vi "py-lv-comm_labview-client_jki-sm.vi"() -> ()   [LabVIEW 2016]
uses:
  <vilib>/addons/zeromq/zmq_context.lvclass
  <vilib>/addons/zeromq/zmq_socket.lvclass
panel:
  in  "Tab Control":enum32{"Python Communication", "Debug"}(tab)
  in  "Stop Server":bool
  in  "Connect to Server":bool
  in  "Send Command":bool
  in  "Command":string
  in  "Wait for response":bool=TRUE
  in  "address":string="tcp://127.0.0.1:15213" caption="TCP address of ZMQ server"
  out "Return string":string
  in  "Read Integer":bool
  in  "Read Double":bool
  in  "Read String":bool
  in  "Read Bool":bool
  in  "Read Numpy Array":bool
  in  "Function":string
  in  "Python Property":bool=TRUE
  in  "Arguments":string[](array[string])
  out "int result":i32
  out "double result":dbl
  out "string result":string
  out "bool result":bool
  out "nparray result":dbl[](array[numeric])
  out "Status":string="Idle"
  in  "OK":bool
  out "error":errorcluster
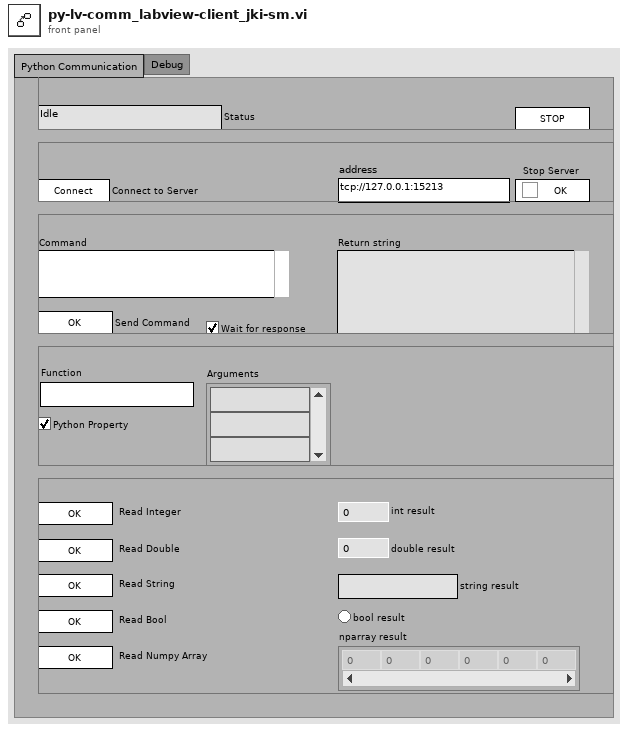
[diagram p1: front panel]
types:
  T1 = enum32{"Invalid", "Standard", "Closed", "Hidden", "Minimized", "Maximized"}
  T2 = enum32{"invalid app kind", "Development System", "Run Time System", "Student Edition", "Embedded LabVIEW", "Evaluation", "Custom"}
  T3 = cluster{"Core":cluster{"Current VI Reference":refnum<vi>, "Close Panel on Exit?":bool}, "zmq_context":refnum<class "zmq_context.lvclass">, "zmq_socket":refnum<class "zmq_socket.lvclass">, "Function":string, "Arguments":string[], "Python Property":bool, "return string":string}
  T4 = cluster{"Current VI Reference":refnum<vi>, "Close Panel on Exit?":bool}
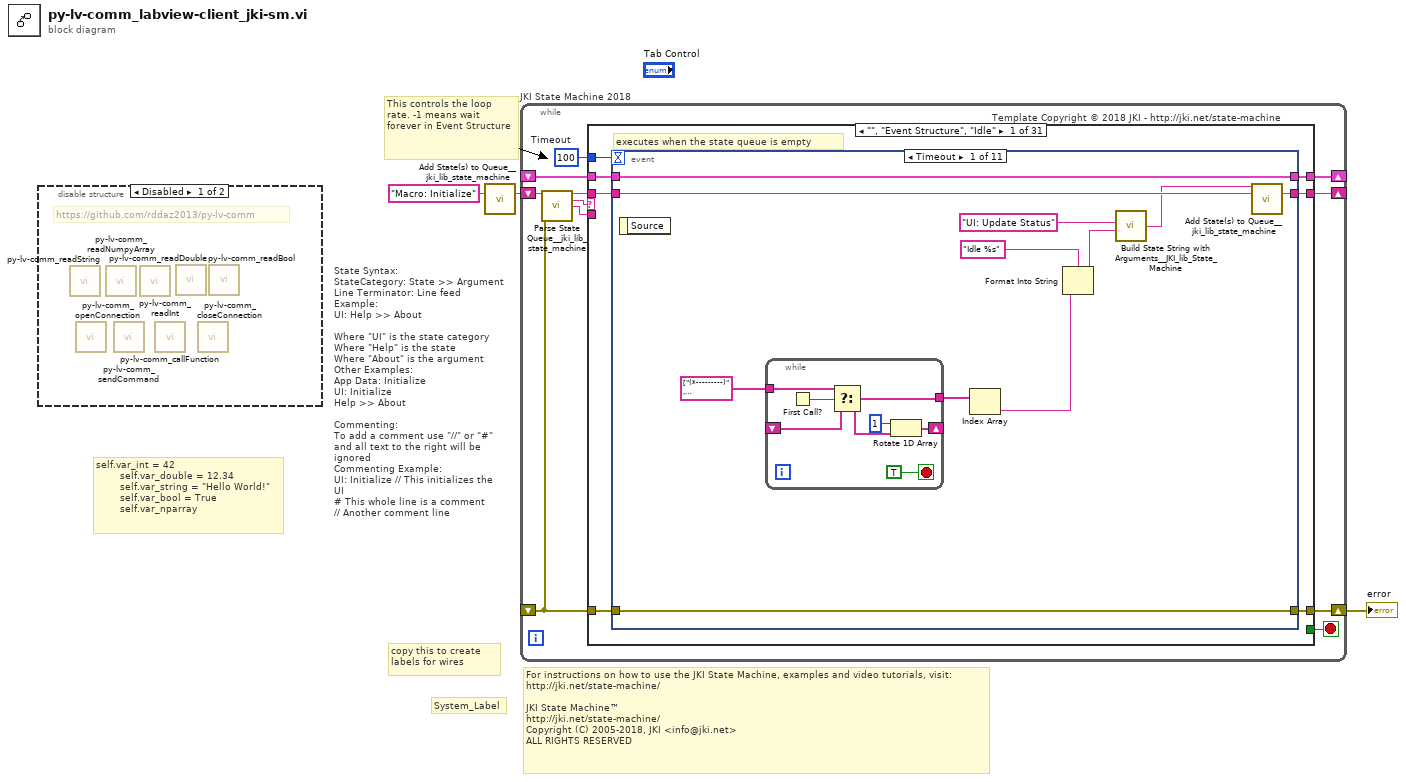
[diagram p0: block diagram]
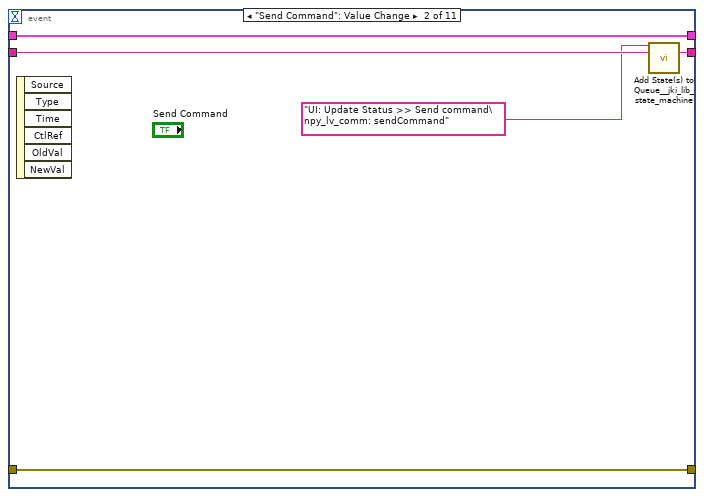
[diagram p3: hidden frame]
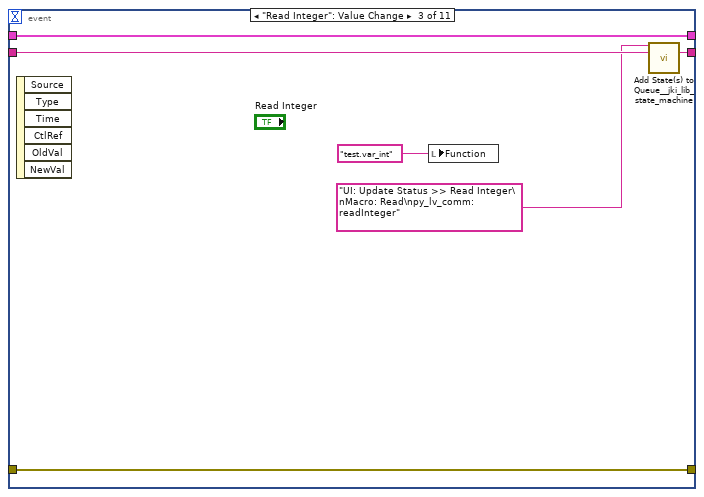
[diagram p4: hidden frame]
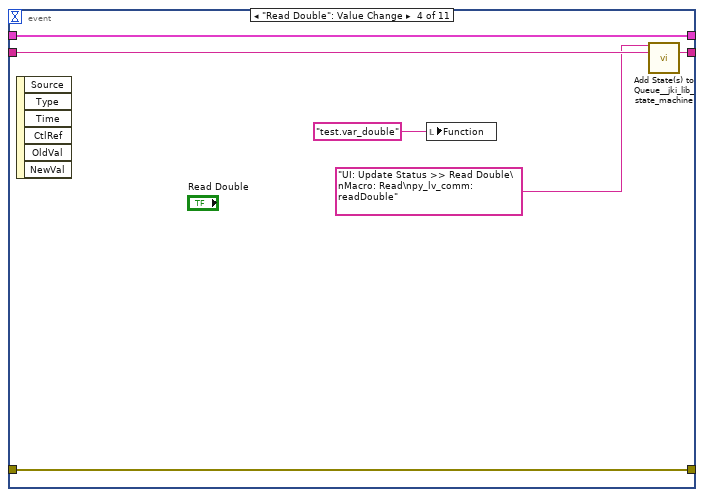
[diagram p5: hidden frame]
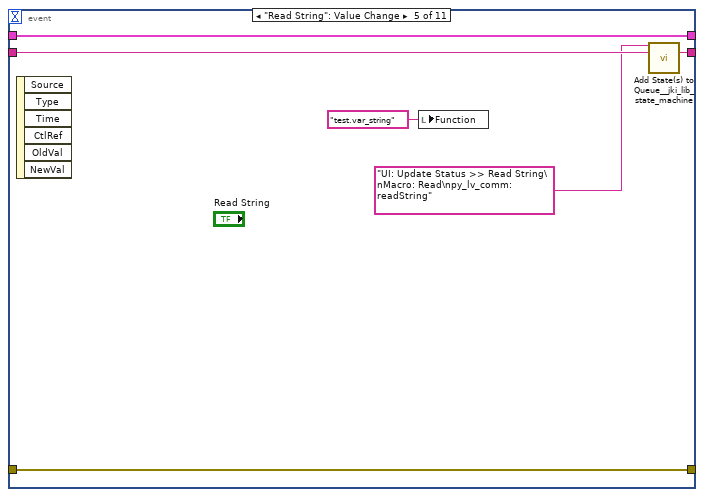
[diagram p6: hidden frame]
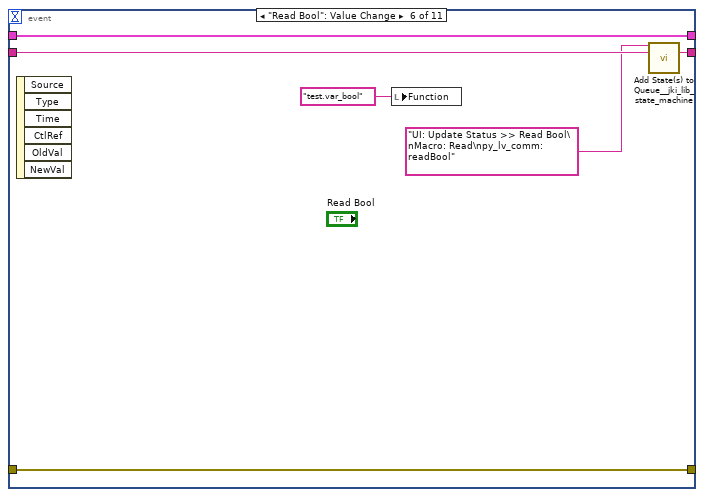
[diagram p7: hidden frame]
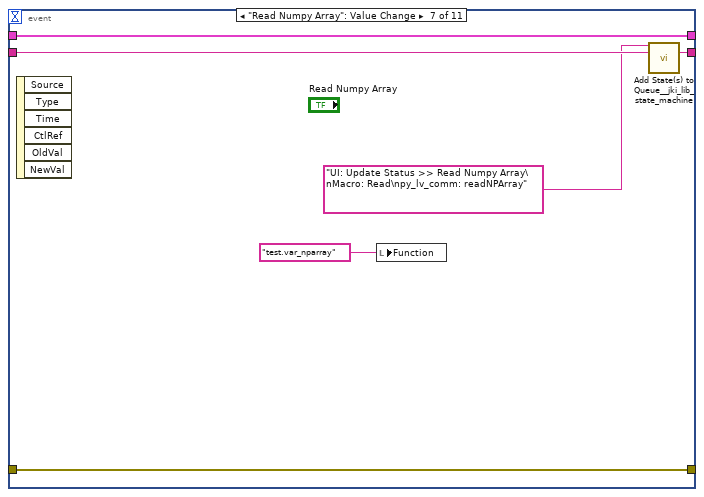
[diagram p8: hidden frame]
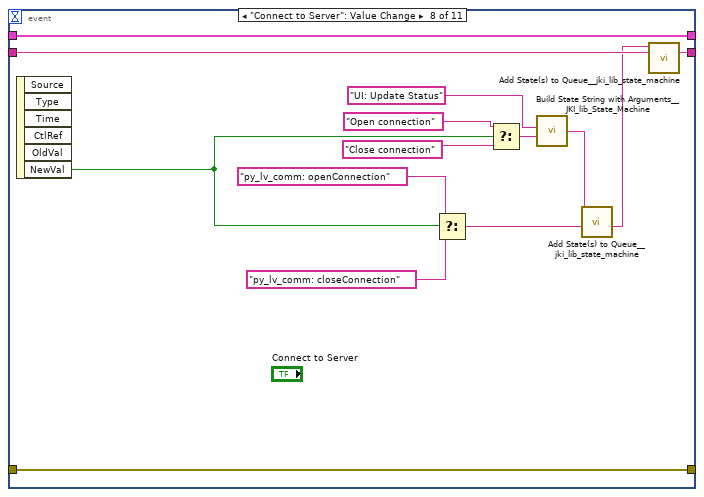
[diagram p9: hidden frame]
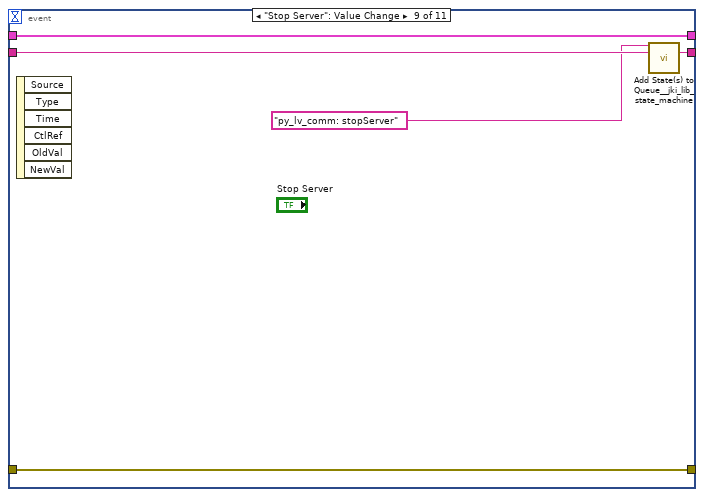
[diagram p10: hidden frame]
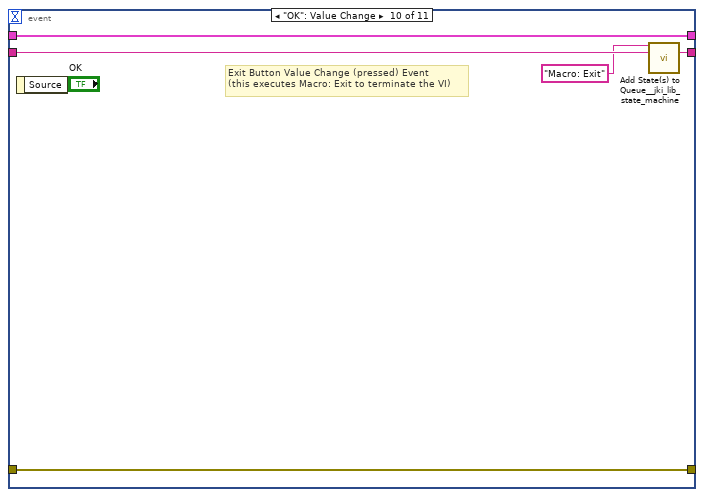
[diagram p11: hidden frame]
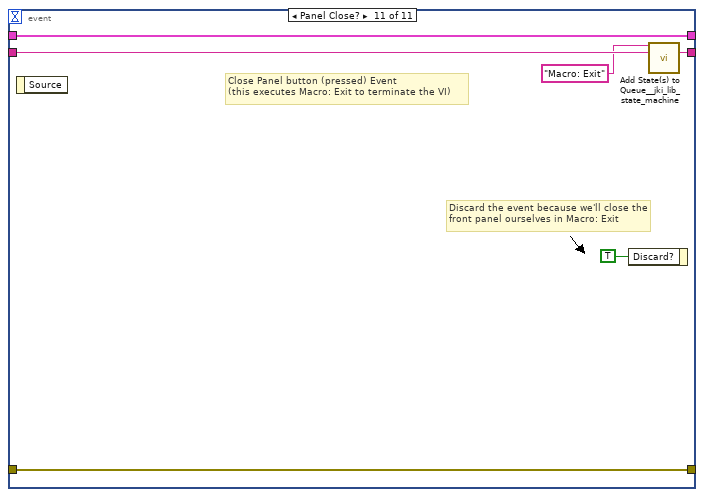
[diagram p12: hidden frame]
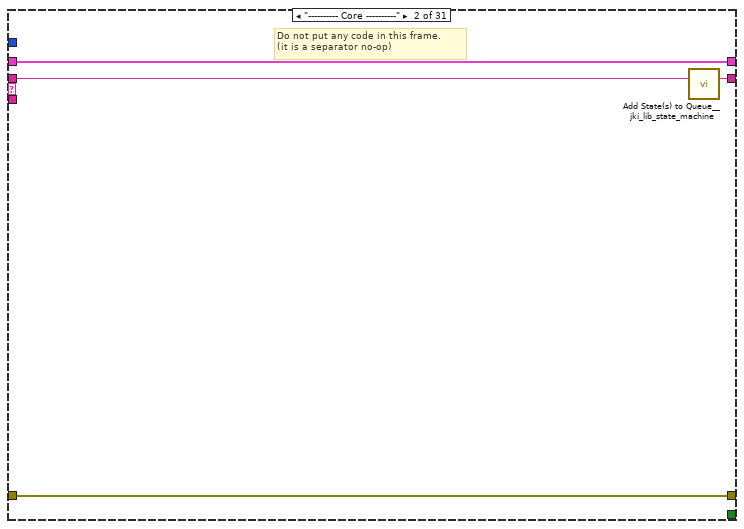
[diagram p13: hidden frame]
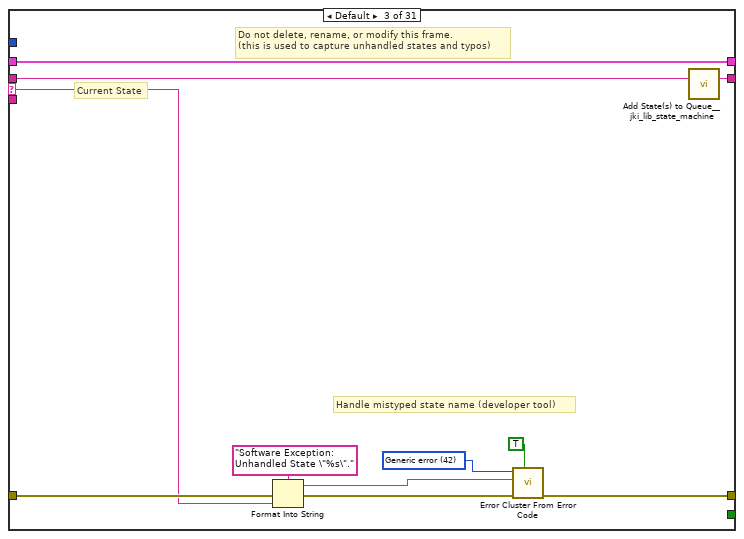
[diagram p14: hidden frame]
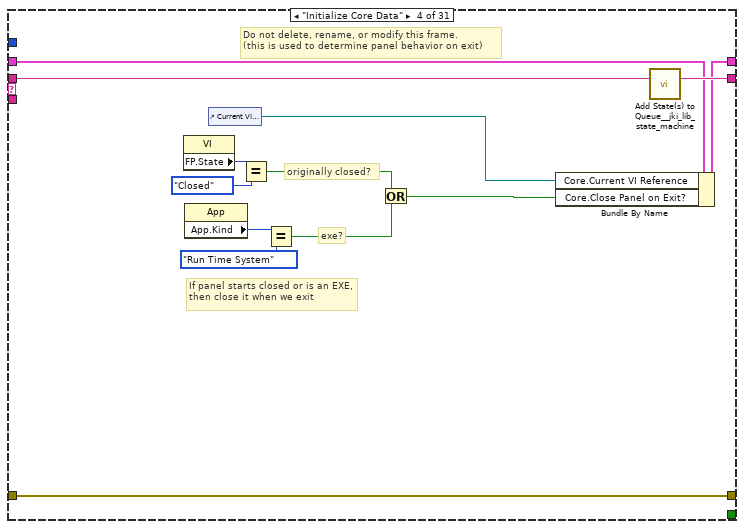
[diagram p15: hidden frame]
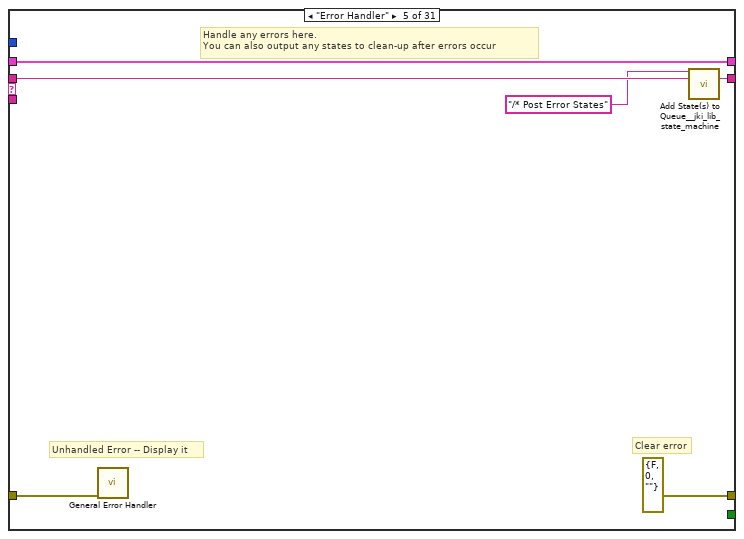
[diagram p16: hidden frame]
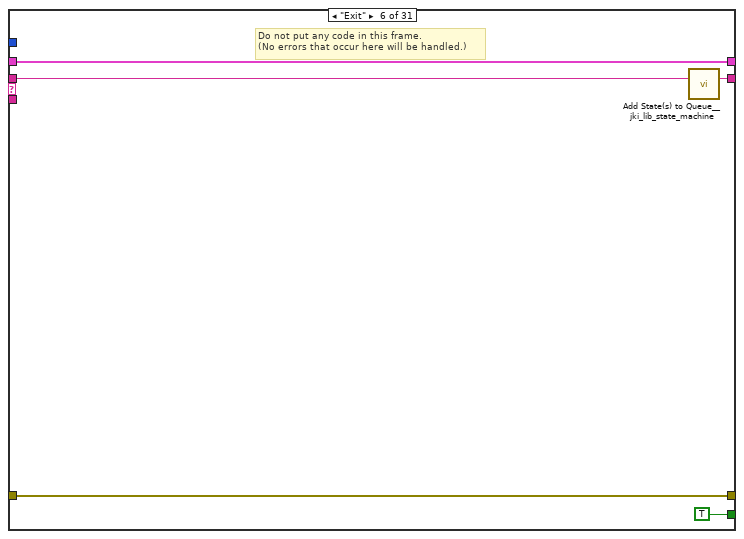
[diagram p17: hidden frame]
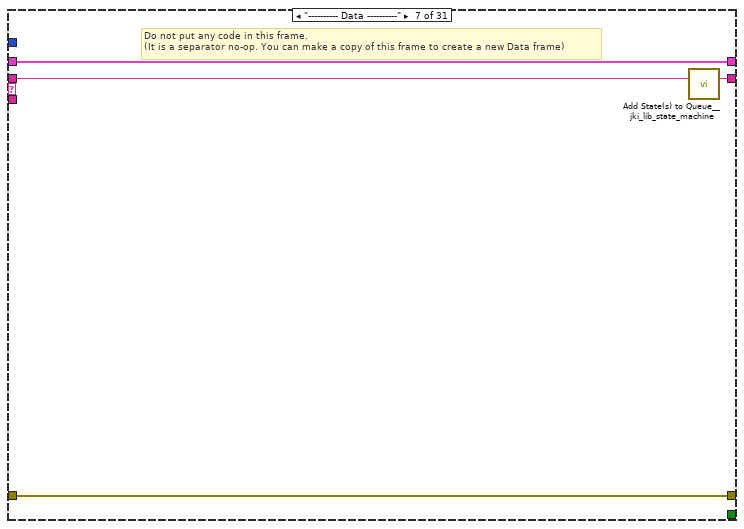
[diagram p18: hidden frame]
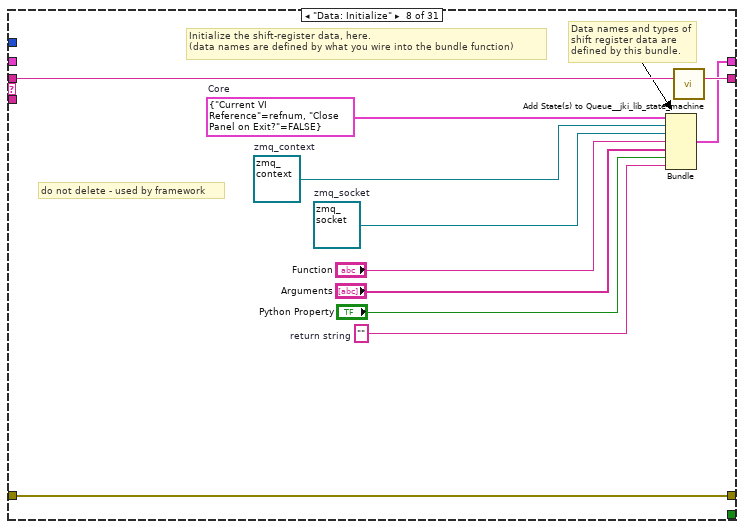
[diagram p19: hidden frame]
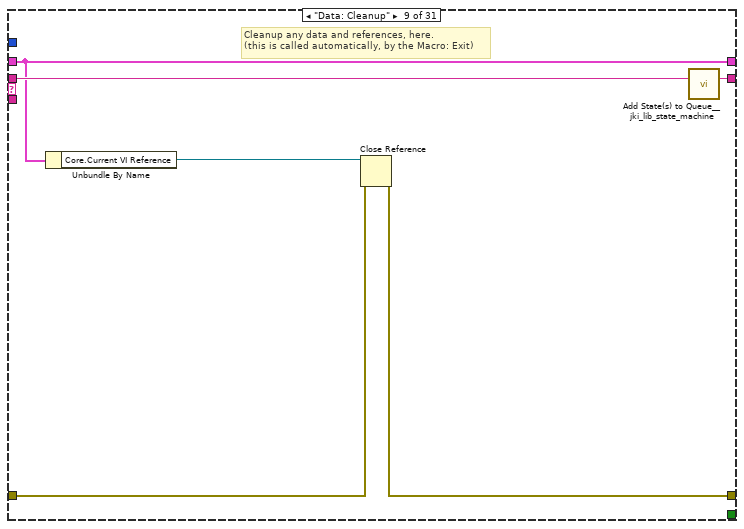
[diagram p20: hidden frame]
diagram:
  # "self.var_int = 42\n        self.var_double = 12.34\n        self.var_string = \"Hello World!\"\n        self.var_bool = True\n        self.var_nparray"
  # "For instructions on how to use the JKI State Machine, examples and video tutorials, visit:\nhttp://jki.net/state-machine/\n\nJKI State Machine™\nhttp://jki.net/state-machine/\nCopyright (C) 2005-2018, JKI <info@jki.net>\nALL RIGHTS RESERVED"
  # "State Syntax:\nStateCategory: State >> Argument\nLine Terminator: Line feed\nExample:\nUI: Help >> About\n\nWhere \"UI\" is the state category\nWhere \"Help\" is the state\nWhere \"About\" is the argument\nOther Examples:\nApp Data: Initialize\nUI: Initialize\nHelp >> About\n\nCommenting:\nTo add a comment use \"//\" or \"#\" and all text to the right will be ignored\nCommenting Example:\nUI: Initialize // This initializes the UI\n# This whole line is a comment\n// Another comment line"
  # "copy this to create labels for wires"
  # "This controls the loop rate. -1 means wait forever in Event Structure"
  # "System_Label"
  n1 = disable-structure shown="Disabled" {
    frame Disabled {
      # "https://github.com/rddaz2013/py-lv-comm"
      n2 = call "py-lv-comm_readString.vi"() -> ()  [unwired: 9 in, 3 out]
      n3 = call "py-lv-comm_openConnection.vi"() -> ()  [unwired: 9 in, 3 out]
      n4 = call "py-lv-comm_readNumpyArray.vi"() -> ()  [unwired: 9 in, 3 out]
      n5 = call "py-lv-comm_sendCommand.vi"() -> ()  [unwired: 9 in, 3 out]
      n6 = call "py-lv-comm_readInt.vi"() -> ()  [unwired: 9 in, 3 out]
      n7 = call "py-lv-comm_callFunction.vi"() -> ()  [unwired: 9 in, 3 out]
      n8 = call "py-lv-comm_readDouble.vi"() -> ()  [unwired: 9 in, 3 out]
      n9 = call "py-lv-comm_closeConnection.vi"() -> ()  [unwired: 11 in, 1 out]
      n10 = call "py-lv-comm_readBool.vi"() -> ()  [unwired: 9 in, 3 out]
    }
    frame Enabled {
    }
  }
  n11 = call <vilib>:"Add State(s) to Queue__jki_lib_state_machine.vi"("State(s) in (\"\")"="Macro: Initialize") -> ("States Out"=w3:string)  [unwired: 14 in]
  n12 = while "JKI State Machine 2018" {
    shift-right: [w7] -> _
    shift-left: _ -> [w6]
    shift-right: [w10] -> w1
    shift-left: _ -> [w4]
    shift-right: [w9] -> _
    shift-left: w3 -> [w11]
    stop <- w8 stop-if-true
    w5 = 100  # Timeout
    # "Template Copyright © 2018 JKI - http://jki.net/state-machine"
    n13 = call <vilib>:"Parse State Queue__jki_lib_state_machine.vi"("State Queue"=w11, "Error In (no error)"=w4) -> ("Remaining States"=w13:string, "Current State"=w14:string, "Arguments"=w12:string)  [unwired: 11 in]
    n14 = case shown="\"\", \"Event Structure\", \"Idle\"" w14 {
      selector: w14 -> [_ _ w108 _ _ _ _ _ _ _ _ _ _ _ _ _ _ _ _ _ _ _ _ _ _ _ _ _ _ _ _]
      tunnel: w13 -> [w21 w107 w112 w131 w137 w142 w146 w157 w163 w171 w175 w180 w185 w190 w196 w207 w276 w281 w286 w296 w300 w309 w322 w338 w345 w358 w367 w376 w385 w394 w404]
      tunnel: w12 -> [_ _ _ _ _ _ _ _ _ _ _ _ w181 _ w191 w201 _ _ _ _ _ _ _ _ _ _ _ _ _ _ _]
      tunnel: w6 -> [w19 w104 w110 w124 w134 w140 w143 _ w158 w165 w172 w178 w182 w187 w194 w203 w273 w278 w283 w293 w297 w304 w318 w329 w341 w349 w364 w373 w382 w391 w402]
      tunnel: [w18 w105 w114 w128 errorcluster {"status"=FALSE, "code"=0, "source"=""} ("error out") w139 w144 w154 w159 w169 w173 w177 w183 w188 w192 w204 w274 w279 w284 w294 w298 w305 w319 w332 w342 w347 w361 w370 w378 w388 w395] -> w10
      tunnel: w4 -> [w17 w105 w113 w128 w133 w139 w144 w154 w160 w169 w173 w177 w183 w188 w193 w205 w274 w279 w284 w294 w298 w306 w320 w333 w343 w354 w359 w368 w380 w386 w396]
      tunnel: [w20 w106 w111 w130 w136 w141 w145 w156 w162 w170 w174 w179 w184 w189 w195 w206 w275 w280 w285 w295 w299 w308 w321 w337 w344 w357 w366 w375 w384 w393 w403] -> w9
      tunnel: [_ _ _ _ _ TRUE _ _ _ _ _ _ _ _ _ _ _ _ _ _ _ _ _ _ _ _ _ _ _ _ _] -> w8
      tunnel: [w16 w104 w110 w129 w134 w140 w143 w155 w158 w164 w172 w178 w182 w187 w194 w203 w273 w278 w283 w293 w297 w303 w317 w328 w341 w348 w364 w373 w382 w391 w402] -> w7
      tunnel: w5 -> [w15 _ _ _ _ _ _ _ _ _ _ _ _ _ _ _ _ _ _ _ _ _ _ _ _ _ _ _ _ _ _]
      frame "", "Event Structure", "Idle" {
        # "executes when the state queue is empty"
        n15 = event shown="[0] Timeout" {
          selector: _ -> [_ _ _ _ _ _ _ _ _ _ _]
          dyn-events: _ -> [_ _ _ _ _ _ _ _ _ _ _]
          timeout: w15 -> [_ _ _ _ _ _ _ _ _ _ _]
          tunnel: w21 -> [w32 w44 w50 w56 w62 w68 w74 w87 w92 w97 w103]
          tunnel: [w31 w43 w49 w55 w61 w67 w73 w86 w91 w96 w102] -> w20
          tunnel: w19 -> [w29 w41 w47 w53 w59 w65 w71 w84 w89 w94 w100]
          tunnel: [w30 w42 w48 w54 w60 w66 w72 w85 w90 w95 w101] -> w18
          tunnel: w17 -> [w30 w42 w48 w54 w60 w66 w72 w85 w90 w95 w101]
          tunnel: [w29 w41 w47 w53 w59 w65 w71 w84 w89 w94 w100] -> w16
          event Timeout {
            n16 = event-data() -> ()  [unwired: 1 in, 1 out]
            n17 = while {
              shift-right: [w35] -> _
              shift-left: _ -> [w36]
              tunnel: string[] ["(*---------)", "(-*--------)", "(--*-------)", "(---*------)", "(----*-----)", "(-----*----)", "(------*---)", "(-------*--)", "(--------*-)", "(---------*)", "(--------*-)", "(-------*--)", "(------*---)", "(-----*----)", "(----*-----)", "(---*------)", "(--*-------)", "(-*--------)"] ("lines") -> [w37]
              tunnel: [w34] -> w27
              stop <- TRUE stop-if-true
              n18 = First Call?() -> (First Call?: T/F=w38:bool)
              n19 = Select(t=w37, s=w38, f=w36) -> (s? t:f=w34:string[])
              n20 = Rotate 1D Array(1:w34, 2:1 ("n")) -> (0:w35:string[])
            }
            n21 = Index Array(array=w27) -> (element=w26:string)  [unwired: 1 in]
            n22 = Format Into String(format string="Idle %s" ("Status"), w26) -> (resulting string=w23:string)  [unwired: 2 in, 1 out]
            n23 = call <vilib>:"Build State String with Arguments__JKI_lib_State_Machine.vi"("Arguments (\"\")"=w23, "State"="UI: Update Status" ("Status")) -> ("State with Arguments"=w22:string)  [unwired: 4 in]
            n24 = call <vilib>:"Add State(s) to Queue__jki_lib_state_machine.vi"("State(s) in Front (\"\")"=w22, "State(s) in (\"\")"=w32) -> ("States Out"=w31:string)  [unwired: 13 in]
          }
          event "Send Command": Value Change {
            n25 = event-data() -> ()  [unwired: 1 in, 6 out]
            n26 = call <vilib>:"Add State(s) to Queue__jki_lib_state_machine.vi"("State(s) in Front (\"\")"="UI: Update Status >> Send command\npy_lv_comm: sendCommand" ("State(s) in Front (\"\")"), "State(s) in (\"\")"=w44) -> ("States Out"=w43:string)  [unwired: 13 in]
          }
          event "Read Integer": Value Change {
            n27 = event-data() -> ()  [unwired: 1 in, 6 out]
            n28 = local write "Function"("test.var_int" ("State(s) in Front (\"\")")) -> ()
            n29 = call <vilib>:"Add State(s) to Queue__jki_lib_state_machine.vi"("State(s) in Front (\"\")"="UI: Update Status >> Read Integer\nMacro: Read\npy_lv_comm: readInteger" ("State(s) in Front (\"\")"), "State(s) in (\"\")"=w50) -> ("States Out"=w49:string)  [unwired: 13 in]
          }
          event "Read Double": Value Change {
            n30 = event-data() -> ()  [unwired: 1 in, 6 out]
            n31 = local write "Function"("test.var_double" ("State(s) in Front (\"\")")) -> ()
            n32 = call <vilib>:"Add State(s) to Queue__jki_lib_state_machine.vi"("State(s) in Front (\"\")"="UI: Update Status >> Read Double\nMacro: Read\npy_lv_comm: readDouble" ("State(s) in Front (\"\")"), "State(s) in (\"\")"=w56) -> ("States Out"=w55:string)  [unwired: 13 in]
          }
          event "Read String": Value Change {
            n33 = event-data() -> ()  [unwired: 1 in, 6 out]
            n34 = local write "Function"("test.var_string" ("State(s) in Front (\"\")")) -> ()
            n35 = call <vilib>:"Add State(s) to Queue__jki_lib_state_machine.vi"("State(s) in Front (\"\")"="UI: Update Status >> Read String\nMacro: Read\npy_lv_comm: readString" ("State(s) in Front (\"\")"), "State(s) in (\"\")"=w62) -> ("States Out"=w61:string)  [unwired: 13 in]
          }
          event "Read Bool": Value Change {
            n36 = event-data() -> ()  [unwired: 1 in, 6 out]
            n37 = local write "Function"("test.var_bool" ("State(s) in Front (\"\")")) -> ()
            n38 = call <vilib>:"Add State(s) to Queue__jki_lib_state_machine.vi"("State(s) in Front (\"\")"="UI: Update Status >> Read Bool\nMacro: Read\npy_lv_comm: readBool" ("State(s) in Front (\"\")"), "State(s) in (\"\")"=w68) -> ("States Out"=w67:string)  [unwired: 13 in]
          }
          event "Read Numpy Array": Value Change {
            n39 = event-data() -> ()  [unwired: 1 in, 6 out]
            n40 = local write "Function"("test.var_nparray" ("State(s) in Front (\"\")")) -> ()
            n41 = call <vilib>:"Add State(s) to Queue__jki_lib_state_machine.vi"("State(s) in Front (\"\")"="UI: Update Status >> Read Numpy Array\nMacro: Read\npy_lv_comm: readNPArray" ("State(s) in Front (\"\")"), "State(s) in (\"\")"=w74) -> ("States Out"=w73:string)  [unwired: 13 in]
          }
          event "Connect to Server": Value Change {
            n42 = event-data() -> ("NewVal"=w79:bool)  [unwired: 1 in, 5 out]
            n43 = Select(t="py_lv_comm: openConnection" ("State(s) in Front (\"\")"), s=w79, f="py_lv_comm: closeConnection" ("State(s) in Front (\"\")")) -> (s? t:f=w78:string)
            n44 = Select(t="Open connection" ("Status"), s=w79, f="Close connection" ("Status")) -> (s? t:f=w77:string)
            n45 = call <vilib>:"Build State String with Arguments__JKI_lib_State_Machine.vi"("Arguments (\"\")"=w77, "State"="UI: Update Status") -> ("State with Arguments"=w76:string)  [unwired: 4 in]
            n46 = call <vilib>:"Add State(s) to Queue__jki_lib_state_machine.vi"("State(s) in Front (\"\")"=w76) -> ()  [unwired: 14 in, 1 out]
            n47 = call <vilib>:"Add State(s) to Queue__jki_lib_state_machine.vi"("State(s) in Front (\"\")"=w78, "State(s) in (\"\")"=w87) -> ("States Out"=w86:string)  [unwired: 13 in]
          }
          event "Stop Server": Value Change {
            n48 = event-data() -> ()  [unwired: 1 in, 6 out]
            n49 = call <vilib>:"Add State(s) to Queue__jki_lib_state_machine.vi"("State(s) in Front (\"\")"="py_lv_comm: stopServer" ("State(s) in Front (\"\")"), "State(s) in (\"\")"=w92) -> ("States Out"=w91:string)  [unwired: 13 in]
          }
          event "OK": Value Change {
            # "Exit Button Value Change (pressed) Event\n(this executes Macro: Exit to terminate the VI)"
            n50 = event-data() -> ()  [unwired: 1 in, 1 out]
            n51 = call <vilib>:"Add State(s) to Queue__jki_lib_state_machine.vi"("State(s) in Front (\"\")"="Macro: Exit", "State(s) in (\"\")"=w97) -> ("States Out"=w96:string)  [unwired: 13 in]
          }
          event Panel Close? {
            # "Discard the event because we'll close the front panel ourselves in Macro: Exit"
            # "Close Panel button (pressed) Event\n(this executes Macro: Exit to terminate the VI)"
            n52 = event-data() -> ()  [unwired: 1 in, 1 out]
            n53 = event-data("Discard?"=TRUE) -> ()  [unwired: 1 in, 1 out]
            n54 = call <vilib>:"Add State(s) to Queue__jki_lib_state_machine.vi"("State(s) in Front (\"\")"="Macro: Exit", "State(s) in (\"\")"=w103) -> ("States Out"=w102:string)  [unwired: 13 in]
          }
        }
      }
      frame "---------- Core ----------" {
        # "Do not put any code in this frame.\n(it is a separator no-op)"
        n55 = call <vilib>:"Add State(s) to Queue__jki_lib_state_machine.vi"("State(s) in (\"\")"=w107) -> ("States Out"=w106:string)  [unwired: 14 in]
      }
      frame Default {
        w117 = 42 items=["No error", "Argument error", "Memory is full", "Out of zone", "End of file", "File already open", "Generic file I/O error", "File not found", "File permission error", "Disk is full", "Duplicate path", "Too many files open", "System feature not enabled", "Resource file not found", "Cannot add resource", "Resource not found", "Image not found", "Image memory error", "Pen does not exist", "Config type invalid", "Config token not found", "Config parse error", "Config memory error", "Bad external code format", "Bad external code offset", "External code not present", "Null window", "Destroy window error", "Null menu", "Print aborted", "Bad print record", "Print driver error", "Windows error during printing", "Memory error during printing", "Print dialog error", "Generic print error", "Invalid device refnum", "Device not found", "Device parameter error", "Device unit error", "Cannot open device", "Device call aborted", "Generic error", "Cancelled by user", "Object ID too low", "Object ID too high", "Object not in heap", "Unknown heap", "Unknown object (invalid DefProc)", "Unknown object (DefProc not in table)", "Message out of range", "Invalid (null) method", "Unknown message", "Manager call not supported", "Bad address", "Network operation in progress", "Network operation timed out", "Connection is busy", "Network attribute not supported", "Network error", "Address in use", "System out of memory", "Connection aborted", "Connection refused", "Not connected", "Already connected", "Connection closed", "Initialization error (interapplication manager)", "Bad occurrence", "Wait on unbound occurrence handler", "Occurrence queue overflow", "Datalog type conflict", "Unused", "Unrecognized type (interapplication manager)", "Memory corrupt", "Failed to make temporary DLL", "Old CIN version", "Drag socket not found", "Failed to load drop-object", "Failed to register OLE object", "Failed to release OLE object", "Format specifier type mismatch", "Unknown format specifier", "Too few format specifiers", "Too many format specifiers", "Scan failed", "Newer CIN version", "Error converting to variant", "Runtime menu error", "Password tampered", "Variant attribute not found", "Incompatible variant data type", "Event data is not available", "Event Store is not present", "Occurrence is not found", "Event Queue is not created", "Event info is not available", "Refnum passed is NULL", "Error retrieving Class GUID", "Error retrieving CoClass GUID", "Error retrieving TypeLib GUID.", "Bad built application magic bytes.", "Specific driver is different from the specific driver associated with the Logical Name.", "There is no session opened to the class driver.", "Max Error", "MAX - Error with config objects", "MAX - Error loading configuration", "MAX - Group not supported"]
        # "Current State"
        # "Do not delete, rename, or modify this frame.\n(this is used to capture unhandled states and typos)"
        # "Handle mistyped state name (developer tool)"
        n56 = Format Into String(format string="Software Exception: Unhandled State \"%s\"." ("message"), error in=w113, w108) -> (resulting string=w116:string, error out=w115:errorcluster)  [unwired: 1 in]
        n57 = call <vilib>:"Error Cluster From Error Code.vi"("show call chain? (False)"=TRUE, "error in (no error)"=w115, "error message (\"\")"=w116, "error code (0)"=w117) -> ("error out"=w114:errorcluster)  [unwired: 5 in]
        n58 = call <vilib>:"Add State(s) to Queue__jki_lib_state_machine.vi"("State(s) in (\"\")"=w112) -> ("States Out"=w111:string)  [unwired: 14 in]
      }
      frame "Initialize Core Data" {
        # "Do not delete, rename, or modify this frame.\n(this is used to determine panel behavior on exit)"
        # "originally closed?"
        # "exe?"
        # "If panel starts closed or is an EXE, then close it when we exit"
        n59 = property class="VI"() -> ("FP.State"=w121:T1)  [unwired: 2 in, 2 out]
        n60 = property class="App"() -> ("App.Kind"=w127:T2)  [unwired: 2 in, 2 out]
        n61 = control-ref of="Current VI Reference"() -> (w122:refnum<vi>)
        n62 = Equal?(x=w121, y=T1."Closed" ("Front Panel Window:State")) -> (x = y?=w119:bool)
        n63 = Equal?(x=w127, y=T2."Run Time System" ("Application:Kind")) -> (x = y?=w125:bool)
        n64 = Or(x=w119, y=w125) -> (x .or. y?=w123:bool)
        n65 = Bundle By Name(cluster=w124, "Core.Current VI Reference"=w122, "Core.Close Panel on Exit?"=w123) -> (w129:T3)
        n66 = call <vilib>:"Add State(s) to Queue__jki_lib_state_machine.vi"("State(s) in (\"\")"=w131) -> ("States Out"=w130:string)  [unwired: 14 in]
      }
      frame "Error Handler" {
        # "Unhandled Error -- Display it"
        # "Handle any errors here.\nYou can also output any states to clean-up after errors occur"
        # "Clear error"
        n67 = call <vilib>:"General Error Handler.vi"("error in (no error)"=w133) -> ()  [unwired: 10 in, 5 out]
        n68 = call <vilib>:"Add State(s) to Queue__jki_lib_state_machine.vi"("State(s) in Front (\"\")"="/* Post Error States", "State(s) in (\"\")"=w137) -> ("States Out"=w136:string)  [unwired: 13 in]
      }
      frame "Exit" {
        # "Do not put any code in this frame.\n(No errors that occur here will be handled.)"
        n69 = call <vilib>:"Add State(s) to Queue__jki_lib_state_machine.vi"("State(s) in (\"\")"=w142) -> ("States Out"=w141:string)  [unwired: 14 in]
      }
      frame "---------- Data ----------" {
        # "Do not put any code in this frame.\n(It is a separator no-op. You can make a copy of this frame to create a new Data frame)"
        n70 = call <vilib>:"Add State(s) to Queue__jki_lib_state_machine.vi"("State(s) in (\"\")"=w146) -> ("States Out"=w145:string)  [unwired: 14 in]
      }
      frame "Data: Initialize" {
        w147 = ""  # return string
        w151 = refnum<class "zmq_socket.lvclass"> refnum  # zmq_socket
        w152 = refnum<class "zmq_context.lvclass"> refnum  # zmq_context
        w153 = T4 {"Current VI Reference"=refnum, "Close Panel on Exit?"=FALSE}  # Core
        # "do not delete - used by framework"
        # "Data names and types of shift register data are defined by this bundle."
        # "Initialize the shift-register data, here.\n(data names are defined by what you wire into the bundle function)"
        n71 = Bundle("Core"=w153, "zmq_context"=w152, "zmq_socket"=w151, "Function"="Function", "Arguments"="Arguments", "Python Property"="Python Property", "return string"=w147) -> (w155:T3)  [unwired: 1 in]
        n72 = call <vilib>:"Add State(s) to Queue__jki_lib_state_machine.vi"("State(s) in (\"\")"=w157) -> ("States Out"=w156:string)  [unwired: 14 in]
      }
      frame "Data: Cleanup" {
        # "Cleanup any data and references, here.\n(this is called automatically, by the Macro: Exit)"
        n73 = Unbundle By Name(w158) -> ("Core.Current VI Reference"=w161:refnum<vi>)
        n74 = Close Reference(reference=w161, error in (no error)=w160) -> (error out=w159:errorcluster)
        n75 = call <vilib>:"Add State(s) to Queue__jki_lib_state_machine.vi"("State(s) in (\"\")"=w163) -> ("States Out"=w162:string)  [unwired: 14 in]
      }
      frame "Data: updateInternalVars" {
        # "Do not put any code in this frame.\n(It is a separator no-op. You can make a copy of this frame to create a new Data frame)"
        n76 = local read "Function"() -> (w168:string)
        n77 = local read "Arguments"() -> (w167:string[])
        n78 = local read "Python Property"() -> (w166:bool)
        n79 = Bundle By Name(cluster=w165, "Function"=w168, "Arguments"=w167, "Python Property"=w166) -> (w164:T3)
        n80 = call <vilib>:"Add State(s) to Queue__jki_lib_state_machine.vi"("State(s) in (\"\")"=w171) -> ("States Out"=w170:string)  [unwired: 14 in]
      }
      frame "---------- UI ----------" {
        # "Do not put any code in this frame.\n(It is a separator no-op. You can make a copy of this frame to create a new UI frame)"
        n81 = call <vilib>:"Add State(s) to Queue__jki_lib_state_machine.vi"("State(s) in (\"\")"=w175) -> ("States Out"=w174:string)  [unwired: 14 in]
      }
      frame "UI: Initialize" {
        # "Initialize the User Interface, here.\n(this is called automatically, by the Macro: Init)"
        n82 = property on="Connect to Server" class="Bool (strict)"("Value"=FALSE ("Connect to Server")) -> ()  [unwired: 2 in, 2 out]
        n83 = call <vilib>:"Add State(s) to Queue__jki_lib_state_machine.vi"("State(s) in (\"\")"=w180) -> ("States Out"=w179:string)  [unwired: 14 in]
      }
      frame "UI: Update Status" {
        # "Do not put any code in this frame.\n(It is a separator no-op. You can make a copy of this frame to create a new UI frame)"
        n84 = call <vilib>:"Add State(s) to Queue__jki_lib_state_machine.vi"("State(s) in (\"\")"=w185) -> ("States Out"=w184:string)  [unwired: 14 in]
        "Status" <- w181
      }
      frame "UI: Update Return Value" {
        # "Do not put any code in this frame.\n(It is a separator no-op. You can make a copy of this frame to create a new UI frame)"
        n85 = Unbundle By Name(w187) -> ("return string"=→"Return string":string)
        n86 = call <vilib>:"Add State(s) to Queue__jki_lib_state_machine.vi"("State(s) in (\"\")"=w190) -> ("States Out"=w189:string)  [unwired: 14 in]
      }
      frame "UI: Cursor Set" {
        # "Argument"
        # "Set and Unset Cursor Busy.\n(Usage: \"UI: Cursor Set >> Busy|Idle\")"
        n87 = case shown="\"Idle\", Default" w191 {
          tunnel: w193 -> [w198 w200]
          tunnel: [w197 w199] -> w192
          frame "Idle", Default {
            n88 = call <vilib>:"Unset Busy.vi"("error in (no error)"=w198) -> ("error out"=w197:errorcluster)  [unwired: 10 in]
          }
          frame "Busy" {
            n89 = call <vilib>:"Set Busy.vi"("error in (no error)"=w200) -> ("error out"=w199:errorcluster)  [unwired: 9 in, 1 out]
          }
        }
        n90 = call <vilib>:"Add State(s) to Queue__jki_lib_state_machine.vi"("State(s) in (\"\")"=w196) -> ("States Out"=w195:string)  [unwired: 14 in]
      }
      frame "UI: Front Panel State" {
        # "Argument"
        # "Set Front Panel Open or Closed\n(Usage: \"UI: Front Panel State >> Open|Close\")"
        n91 = Unbundle By Name(w203) -> ("Core.Current VI Reference"=w202:refnum<vi>)
        n92 = case shown="\"Minimize\", \"Minimized\"" w201 {
          tunnel: w205 -> [w213 w228 w239 w252 w265]
          tunnel: [w215 w229 w241 w254 w267] -> w204
          tunnel: w202 -> [w214 w226 w240 w253 w266]
          frame "Open", "Standard", Default {
            w208 = T1."Standard" ("State")
            n93 = property class="VI"(reference=w214, error in=w213) -> (reference out=w211:refnum<vi>, error out=w212:errorcluster, "FP.State"=w210:T1)
            n94 = Not Equal?(x=w210, y=w208) -> (x != y?=w209:bool)
            n95 = case shown="True" w209 {
              tunnel: [w219 w221] -> w215
              tunnel: w212 -> [w218 w221]
              tunnel: w211 -> [w217 _]
              tunnel: w208 -> [w216 _]
              frame True {
                n96 = invoke class="VI" method="FP.Open"(reference=w217, error in=w218, "Activate"=TRUE, "State"=w216) -> (error out=w219:errorcluster)  [unwired: 1 in, 4 out]
              }
              frame False {
              }
            }
          }
          frame "Close", "Closed" {
            n97 = property class="VI"(reference=w226, error in=w228) -> (reference out=w225:refnum<vi>, error out=w227:errorcluster, "FP.State"=w223:T1)
            n98 = Not Equal?(x=w223, y=T1."Closed" ("Front Panel Window:State")) -> (x != y?=w222:bool)
            n99 = case shown="True" w222 {
              tunnel: [w230 w233] -> w229
              tunnel: w227 -> [w230 w232]
              tunnel: w225 -> [_ w231]
              frame False {
              }
              frame True {
                n100 = invoke class="VI" method="FP.Close"(reference=w231, error in=w232) -> (error out=w233:errorcluster)  [unwired: 1 in, 2 out]
              }
            }
          }
          frame "Hidden", "Hide" {
            w234 = T1."Hidden" ("State")
            n101 = property class="VI"(reference=w240, error in=w239) -> (reference out=w237:refnum<vi>, error out=w238:errorcluster, "FP.State"=w236:T1)
            n102 = Not Equal?(x=w236, y=w234) -> (x != y?=w235:bool)
            n103 = case shown="True" w235 {
              tunnel: [w245 w246] -> w241
              tunnel: w238 -> [w244 w246]
              tunnel: w237 -> [w243 _]
              tunnel: w234 -> [w242 _]
              frame True {
                n104 = invoke class="VI" method="FP.Open"(reference=w243, error in=w244, "State"=w242) -> (error out=w245:errorcluster)  [unwired: 2 in, 4 out]
              }
              frame False {
              }
            }
          }
          frame "Minimize", "Minimized" {
            w247 = T1."Minimized" ("State")
            n105 = property class="VI"(reference=w253, error in=w252) -> (reference out=w250:refnum<vi>, error out=w251:errorcluster, "FP.State"=w249:T1)
            n106 = Not Equal?(x=w249, y=w247) -> (x != y?=w248:bool)
            n107 = case shown="True" w248 {
              tunnel: [w258 w259] -> w254
              tunnel: w251 -> [w257 w259]
              tunnel: w250 -> [w256 _]
              tunnel: w247 -> [w255 _]
              frame True {
                n108 = invoke class="VI" method="FP.Open"(reference=w256, error in=w257, "State"=w255) -> (error out=w258:errorcluster)  [unwired: 2 in, 4 out]
              }
              frame False {
              }
            }
          }
          frame "Maximize", "Maximized" {
            w260 = T1."Maximized" ("State")
            n109 = property class="VI"(reference=w266, error in=w265) -> (reference out=w263:refnum<vi>, error out=w264:errorcluster, "FP.State"=w262:T1)
            n110 = Not Equal?(x=w262, y=w260) -> (x != y?=w261:bool)
            n111 = case shown="True" w261 {
              tunnel: [w271 w272] -> w267
              tunnel: w264 -> [w270 w272]
              tunnel: w263 -> [w269 _]
              tunnel: w260 -> [w268 _]
              frame True {
                n112 = invoke class="VI" method="FP.Open"(reference=w269, error in=w270, "State"=w268) -> (error out=w271:errorcluster)  [unwired: 2 in, 4 out]
              }
              frame False {
              }
            }
          }
        }
        n113 = call <vilib>:"Add State(s) to Queue__jki_lib_state_machine.vi"("State(s) in (\"\")"=w207) -> ("States Out"=w206:string)  [unwired: 14 in]
      }
      frame "---------- Macro ----------" {
        # "Do not put any code in this frame.\n(It is a separator no-op. You can make a copy of this frame to create a new Macro frame)"
        n114 = call <vilib>:"Add State(s) to Queue__jki_lib_state_machine.vi"("State(s) in (\"\")"=w276) -> ("States Out"=w275:string)  [unwired: 14 in]
      }
      frame "Macro: Initialize" {
        w277 = "Data: Initialize\nInitialize Core Data\nUI: Initialize\nUI: Front Panel State >> Open"  # Data: Initialize Initialize Core Data UI: Initialize UI: Front Panel State >> Open
        # "Initialization Macro\n(This is called once, when the VI starts)"
        n115 = call <vilib>:"Add State(s) to Queue__jki_lib_state_machine.vi"("State(s) in Front (\"\")"=w277, "State(s) in (\"\")"=w281) -> ("States Out"=w280:string)  [unwired: 13 in]
      }
      frame "Macro: Read" {
        # "Do not put any code in this frame.\n(It is a separator no-op. You can make a copy of this frame to create a new Macro frame)"
        n116 = call <vilib>:"Add State(s) to Queue__jki_lib_state_machine.vi"("State(s) in Front (\"\")"="Data: updateInternalVars\npy_lv_comm: callFunction\nUI: Update Return Value" ("State(s) in Front (\"\")"), "State(s) in (\"\")"=w286) -> ("States Out"=w285:string)  [unwired: 13 in]
      }
      frame "Macro: Exit" {
        # "Exit Macro\n(This is called once, when the VI exits)"
        n117 = Unbundle By Name(w293) -> ("Core.Close Panel on Exit?"=w292:bool)
        n118 = Select(t="UI: Front Panel State >> Close", s=w292, f="") -> (s? t:f=w289:string)
        n119 = call <vilib>:"Add State(s) to Queue__jki_lib_state_machine.vi"("State(s) in (\"\")"=w289, "State(s) at Back (\"\")"="py_lv_comm: closeConnection\nData: Cleanup\nExit") -> ("States Out"=w287:string)  [unwired: 13 in]
        n120 = call <vilib>:"Add State(s) to Queue__jki_lib_state_machine.vi"("State(s) in Front (\"\")"=w287, "State(s) in (\"\")"=w296) -> ("States Out"=w295:string)  [unwired: 13 in]
      }
      frame "---------- py_lv_comm ----------" {
        # "Template Separator\n(You can make a copy of, or modify, this frame)"
        n121 = call <vilib>:"Add State(s) to Queue__jki_lib_state_machine.vi"("State(s) in (\"\")"=w300) -> ("States Out"=w299:string)  [unwired: 14 in]
      }
      frame "py_lv_comm: openConnection" {
        # "Template Separator\n(You can make a copy of, or modify, this frame)"
        n122 = call "py-lv-comm_openConnection.vi"("error in"=w306, "TCP address"="address") -> ("error out"=w305:errorcluster, "socket out"=w301:refnum<class "zmq_socket.lvclass">, "zmq_context out"=w307:refnum<class "zmq_context.lvclass">)  [unwired: 7 in]
        n123 = Bundle By Name(cluster=w304, "zmq_context"=w307, "zmq_socket"=w301) -> (w303:T3)
        n124 = call <vilib>:"Add State(s) to Queue__jki_lib_state_machine.vi"("State(s) in (\"\")"=w309) -> ("States Out"=w308:string)  [unwired: 14 in]
      }
      frame "py_lv_comm: closeConnection" {
        w315 = refnum<class "zmq_socket.lvclass"> refnum ("zmq_socket")
        w316 = refnum<class "zmq_context.lvclass"> refnum ("zmq_context")
        # "Template Separator\n(You can make a copy of, or modify, this frame)"
        n125 = Unbundle By Name(w318) -> ("zmq_context"=w311:refnum<class "zmq_context.lvclass">, "zmq_socket"=w310:refnum<class "zmq_socket.lvclass">)
        n126 = Equal?(x=w316, y=w311) -> (x = y?=w313:bool)
        n127 = Equal?(x=w315, y=w310) -> (x = y?=w314:bool)
        n128 = Or(x=w313, y=w314) -> (x .or. y?=w312:bool)
        n129 = case shown="False" w312 {
          tunnel: w320 -> [w326 w327]
          tunnel: [w325 w327] -> w319
          tunnel: w311 -> [w324 _]
          tunnel: w310 -> [w323 _]
          frame False {
            n130 = call "py-lv-comm_closeConnection.vi"("error in (no error)"=w326, "socket in"=w323, "zmq_context in"=w324) -> ("error out"=w325:errorcluster)  [unwired: 8 in]
          }
          frame True {
          }
        }
        n131 = Bundle By Name(cluster=w318, "zmq_context"=w316, "zmq_socket"=w315) -> (w317:T3)
        n132 = call <vilib>:"Add State(s) to Queue__jki_lib_state_machine.vi"("State(s) in (\"\")"=w322) -> ("States Out"=w321:string)  [unwired: 14 in]
      }
      frame "py_lv_comm: sendCommand" {
        # "Your code here.\n(You can make a copy of, or modify, this frame)"
        n133 = Unbundle By Name(w329) -> ("zmq_socket"=w335:refnum<class "zmq_socket.lvclass">)
        n134 = local write "Send Command"(FALSE ("Send Command")) -> ()
        n135 = call "py-lv-comm_sendCommand.vi"("Wait for response (T)"="Wait for response", "error in (no error)"=w333, "command"="Command", "zmq_socket in"=w335) -> ("error out"=w332:errorcluster, "data"=w330:string)  [unwired: 5 in, 1 out]
        n136 = Bundle By Name(cluster=w329, "return string"=w330) -> (w328:T3)
        n137 = call <vilib>:"Add State(s) to Queue__jki_lib_state_machine.vi"("State(s) in (\"\")"=w338) -> ("States Out"=w337:string)  [unwired: 14 in]
      }
      frame "py_lv_comm: stopServer" {
        # "Template Separator\n(You can make a copy of, or modify, this frame)"
        n138 = Unbundle By Name(w341) -> ("zmq_socket"=w340:refnum<class "zmq_socket.lvclass">)
        n139 = call "py-lv-comm_sendCommand.vi"("error in (no error)"=w343, "command"="exit()", "zmq_socket in"=w340) -> ("error out"=w342:errorcluster)  [unwired: 6 in, 2 out]
        n140 = call <vilib>:"Add State(s) to Queue__jki_lib_state_machine.vi"("State(s) in (\"\")"=w345) -> ("States Out"=w344:string)  [unwired: 14 in]
      }
      frame "py_lv_comm: callFunction" {
        # "Template Separator\n(You can make a copy of, or modify, this frame)"
        n141 = Unbundle By Name(w349) -> ("Python Property"=w353:bool, "zmq_socket"=w356:refnum<class "zmq_socket.lvclass">, "Function"=w351:string, "Arguments"=w352:string[])
        n142 = local write "Read Integer"(FALSE ("Read Integer")) -> ()
        n143 = call "py-lv-comm_callFunction.vi"("Wait for response (T)"=TRUE, "Property (F)"=w353, "error in (no error)"=w354, "arguments"=w352, "function"=w351, "zmq_socket in"=w356) -> ("error out"=w347:errorcluster, "return value"=w350:string)  [unwired: 3 in, 1 out]
        n144 = Bundle By Name(cluster=w349, "return string"=w350) -> (w348:T3)
        n145 = call <vilib>:"Add State(s) to Queue__jki_lib_state_machine.vi"("State(s) in (\"\")"=w358) -> ("States Out"=w357:string)  [unwired: 14 in]
      }
      frame "py_lv_comm: readInteger" {
        # "Template Separator\n(You can make a copy of, or modify, this frame)"
        n146 = Unbundle By Name(w364) -> ("return string"=w360:string)
        n147 = local write "Read Integer"(FALSE ("Read Integer")) -> ()
        n148 = Unflatten From JSON(JSON string=w360, type and defaults=0, error in (no error)=w359) -> (value=→"int result":i32, error out=w361:errorcluster)  [unwired: 4 in]
        n149 = call <vilib>:"Add State(s) to Queue__jki_lib_state_machine.vi"("State(s) in (\"\")"=w367) -> ("States Out"=w366:string)  [unwired: 14 in]
      }
      frame "py_lv_comm: readDouble" {
        # "Template Separator\n(You can make a copy of, or modify, this frame)"
        n150 = Unbundle By Name(w373) -> ("return string"=w369:string)
        n151 = Unflatten From JSON(JSON string=w369, type and defaults=0.0, error in (no error)=w368) -> (value=→"double result":dbl, error out=w370:errorcluster)  [unwired: 4 in]
        n152 = local write "Read Double"(FALSE ("Read Integer")) -> ()
        n153 = call <vilib>:"Add State(s) to Queue__jki_lib_state_machine.vi"("State(s) in (\"\")"=w376) -> ("States Out"=w375:string)  [unwired: 14 in]
      }
      frame "py_lv_comm: readString" {
        # "Template Separator\n(You can make a copy of, or modify, this frame)"
        n154 = Unbundle By Name(w382) -> ("return string"=w381:string)
        n155 = Unflatten From JSON(JSON string=w381, type and defaults="", error in (no error)=w380) -> (value=→"string result":string, error out=w378:errorcluster)  [unwired: 4 in]
        n156 = local write "Read String"(FALSE ("Read Integer")) -> ()
        n157 = call <vilib>:"Add State(s) to Queue__jki_lib_state_machine.vi"("State(s) in (\"\")"=w385) -> ("States Out"=w384:string)  [unwired: 14 in]
      }
      frame "py_lv_comm: readBool" {
        # "Template Separator\n(You can make a copy of, or modify, this frame)"
        n158 = Unbundle By Name(w391) -> ("return string"=w390:string)
        n159 = Unflatten From JSON(JSON string=w390, type and defaults=TRUE, error in (no error)=w386) -> (value=→"bool result":bool, error out=w388:errorcluster)  [unwired: 4 in]
        n160 = local write "Read Bool"(FALSE ("Read Integer")) -> ()
        n161 = call <vilib>:"Add State(s) to Queue__jki_lib_state_machine.vi"("State(s) in (\"\")"=w394) -> ("States Out"=w393:string)  [unwired: 14 in]
      }
      frame "py_lv_comm: readNPArray" {
        # "Template Separator\n(You can make a copy of, or modify, this frame)"
        n162 = Unbundle By Name(w402) -> ("return string"=w401:string)
        n163 = Unflatten From JSON(path=string[] ["__ndarray__"], JSON string=w401, type and defaults=dbl[] [], error in (no error)=w396) -> (value=→"nparray result":dbl[], error out=w395:errorcluster)  [unwired: 3 in]
        n164 = local write "Read Numpy Array"(FALSE ("Read Integer")) -> ()
        n165 = call <vilib>:"Add State(s) to Queue__jki_lib_state_machine.vi"("State(s) in (\"\")"=w404) -> ("States Out"=w403:string)  [unwired: 14 in]
      }
    }
  }
  "error" <- w1
